vi "KalmanFilterLatencyComp_Reset.vi"(11 "inKalmanFilterLatencyCompensator":T1) -> (3 "outKalmanFilterLatencyCompensator":T1)   [LabVIEW 2019, in "Trajectory_Library.lvlib"]
doc: "Creates a new LINEAR SYSTEM data cluster with the specified values. \n\n\nInputs: \n - XXX -- XXX.\n\nOutputs:\n - XXX -- XXX."
uses:
  OBSERVER_SNAP_LIST_ITEM.ctl
  OBSERVER_SNAPSHOT.ctl
  <vilib>/Analysis/Matrix/Datatypes/RealMatrix.ctl
  Trajectory_Library.lvlib
  <vilib>/Analysis/Matrix/NI_Matrix.lvlib
  KALMAN_FILTER_LATENCY_COMP.ctl
panel:
  # "<Statess,1>"
  # "<States, States>"
  # "<Inputs, 1>"
  # "<Outputs,  1>"
  # "<Statess,1>"
  # "<States, States>"
  # "<Inputs, 1>"
  # "<Outputs,  1>"
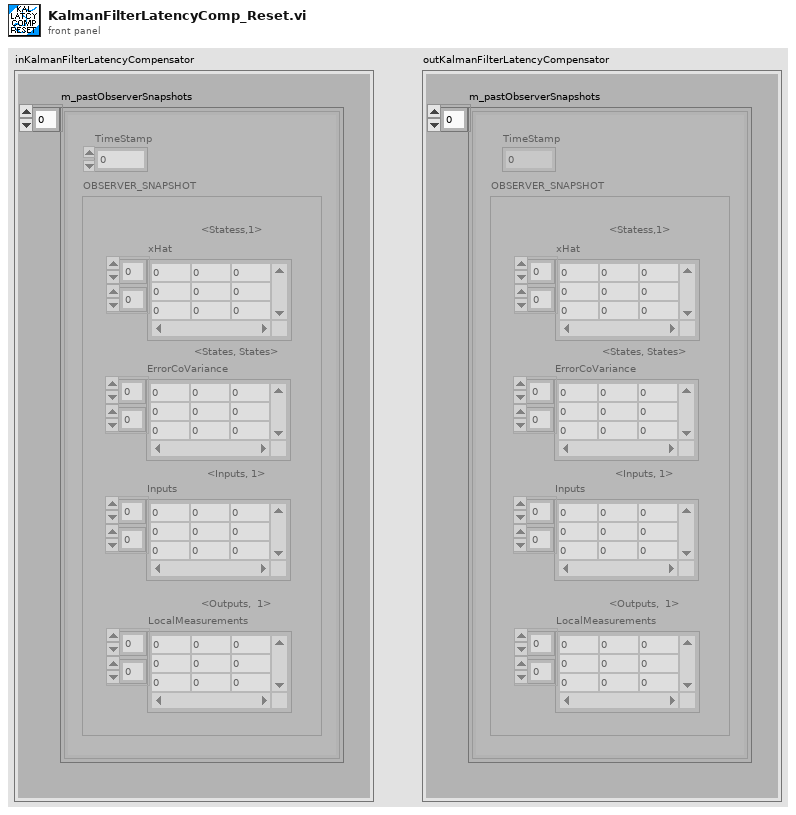
[diagram p1: front panel]
types:
  T1 = typedef "Trajectory_Library.lvlib/KALMAN_FILTER_LATENCY_COMP.ctl" = cluster{"m_pastObserverSnapshots ":T2[]}
  T2 = typedef "Trajectory_Library.lvlib/OBSERVER_SNAP_LIST_ITEM.ctl" = cluster{"TimeStamp":dbl, "OBSERVER_SNAPSHOT":T3}
  T3 = typedef "Trajectory_Library.lvlib/OBSERVER_SNAPSHOT.ctl" = cluster{"ErrorCoVariance":T4, "xHat":T4, "LocalMeasurements":T4, "Inputs":T4}
  T4 = typedef "NI_Matrix.lvlib/RealMatrix.ctl" = dbl[][]
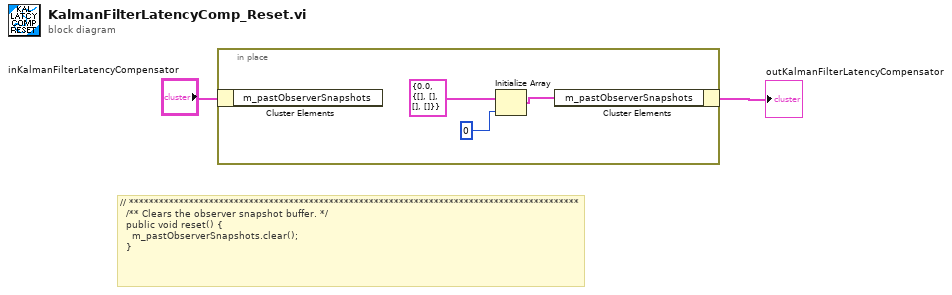
[diagram p0: block diagram]
diagram:
  # "// ******************************************************************************************\n  /** Clears the observer snapshot buffer. */\n  public void reset() {\n    m_pastObserverSnapshots.clear();\n  }"
  n1 = in-place {
    n2 = in-place-cluster #1("inKalmanFilterLatencyCompensator") -> ()  [unwired: 1 out]
    n3 = Initialize Array(T2 {"TimeStamp"=0.0, "OBSERVER_SNAPSHOT"={"ErrorCoVariance"=[], "xHat"=[], "LocalMeasurements"=[], "Inputs"=[]}} ("OBSERVER_LIST_ITEM"), 0 ("dimension size")) -> (w3:T2[])
    n4 = in-place-cluster #1("m_pastObserverSnapshots"=w3) -> (→"outKalmanFilterLatencyCompensator":T1)
  }
